vi "XY graph cursor.vi"() -> ()   [LabVIEW 2020]
uses:
  <vilib>/Utility/miscctls.llb/LVCursorListTypeDef.ctl
panel:
  out "Cursor List 2":T1
  out "Waveform Graph for reference":dbl[](graph)
  in  "Cursor List":T1=[{"Name"="", "Color"=0, "Style"=0, "Point Style"=0, "Name Visible"=TRUE, "Allow Drag"=FALSE, "Cursor Mode"=0, "Plot"=0, "Index"=0, "Position"={"X"=0.0, "Y"=0.0}, "X Scale"=0, "Y Scale"=0, "Watch Plots"=[], "Watch All Plots"=FALSE, "Plot Area"=0, "Label Offset"={"X"=8.0, "Y"=0.05}}]
  out "XY Graph":cluster{i32, "number: 0 to 1":dbl}[](graph)
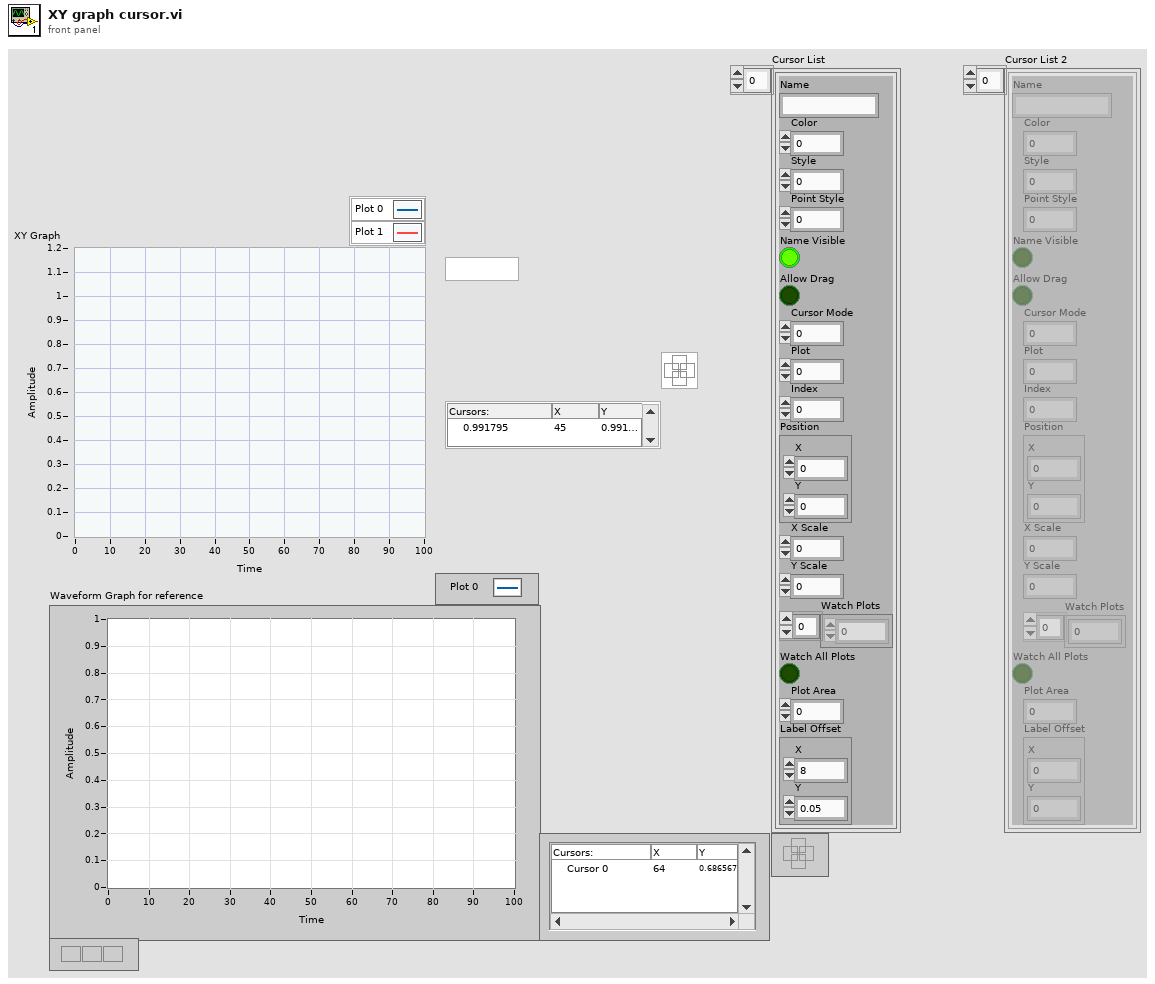
[diagram p1: front panel]
types:
  T1 = typedef "LVCursorListTypeDef.ctl" = cluster{"Name":string, "Color":u32, "Style":u8, "Point Style":u8, "Name Visible":bool, "Allow Drag":bool, "Cursor Mode":u32, "Plot":i32, "Index":i32, "Position":cluster{"X":dbl, "Y":dbl}, "X Scale":u32, "Y Scale":u32, "Watch Plots":i32[], "Watch All Plots":bool, "Plot Area":i32, "Label Offset":cluster{"X":dbl, "Y":dbl}}[]
  T2 = cluster{"Name":string, "Color":u32, "Style":u8, "Point Style":u8, "Name Visible":bool, "Allow Drag":bool, "Cursor Mode":u32, "Plot":i32, "Index":i32, "Position":cluster{"X":dbl, "Y":dbl}, "X Scale":u32, "Y Scale":u32, "Watch Plots":i32[], "Watch All Plots":bool, "Plot Area":i32, "Label Offset":cluster{"X":dbl, "Y":dbl}}
  T3 = cluster{"Name":string, "Color":u32, "Style":u8, "Point Style":u8, "Name Visible":bool, "Allow Drag":bool, "Cursor Mode":u32, "Plot":i32, "Index":i32, "Position":cluster{"X":dbl, "Y":dbl}, "X Scale":u32, "Y Scale":u32, "Watch Plots":i32[], "Watch All Plots":bool, "Plot Area":i32, "Label Offset":cluster{"X":dbl, "Y":dbl}}[]
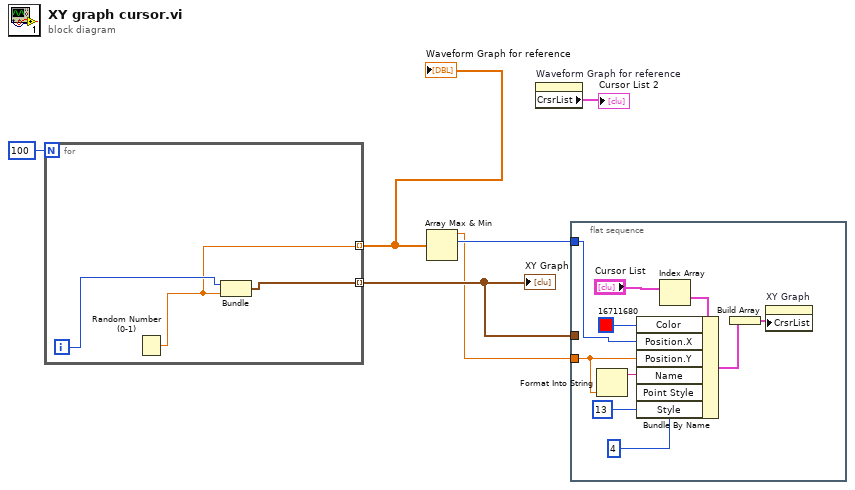
[diagram p0: block diagram]
diagram:
  n1 = for {
    N: 100 -> [_]
    tunnel: [w9] -> w5 mode=indexing
    tunnel: [w7] -> w2 mode=indexing
    i -> [w8]
    n2 = Random Number (0-1)() -> (number: 0 to 1=w7:dbl)
    n3 = Bundle(w8, "number: 0 to 1"=w7) -> (w9:cluster{i32, "number: 0 to 1":dbl})  [unwired: 1 in]
  }
  "XY Graph" <- w5
  "Waveform Graph for reference" <- w2
  n4 = Array Max & Min(array=w2) -> (max value=w3:dbl, max index (indices)=w4:i32)  [unwired: 2 out]
  n5 = property on="Waveform Graph for reference" class="WFGraph (strict)"() -> ("CrsrList"=→"Cursor List 2":T1)  [unwired: 2 in, 2 out]
  n6 = flat-sequence {
    tunnel: w5 -> [_]
    tunnel: w4 -> [w14]
    tunnel: w3 -> [w12]
    frame #0 {
      n7 = Format Into String(w12) -> (resulting string=w13:string)  [unwired: 3 in, 1 out]
      n8 = Index Array(array="Cursor List") -> (element=w18:T2)  [unwired: 1 in]
      n9 = Bundle By Name(cluster=w18, "Color"=u32 16711680, "Position.X"=w14, "Position.Y"=w12, "Name"=w13, "Point Style"=u8 13, "Style"=u8 4) -> (w17:T2)
      n10 = Build Array(w17) -> (w16:T3)
      n11 = property on="XY Graph" class="XYGraph (strict)"("CrsrList"=w16) -> ()  [unwired: 2 in, 2 out]
    }
  }
